vi "Packet.vi"(8 "error in (no error)":errorcluster, 9 "timeout ms (10000)":i32=10000, 11 "connection ID":refnum<k5>) -> (0 "error out":errorcluster, 1 "tx":T1, 2 "px":T2 {"Px16" format="%.2f"; "Px15" format="%.2f"; "Px14" format="%.2f"; "Px13" format="%.2f"; "Px12" format="%.2f"; "Px11" format="%.2f"; "Px10" format="%.2f"; "Px9" format="%.2f"; "Px8" format="%.2f"; "Px7" format="%.2f"; "Px6" format="%.2f"; "Px5" format="%.2f"; "Px4" format="%.2f"; "Px3" format="%.2f"; "Px2" format="%.2f"; "Px1" format="%.2f"}, 3 "connection ID out":refnum<k5>, 4 "frame":u32, 5 "status":string)   [LabVIEW 2019]
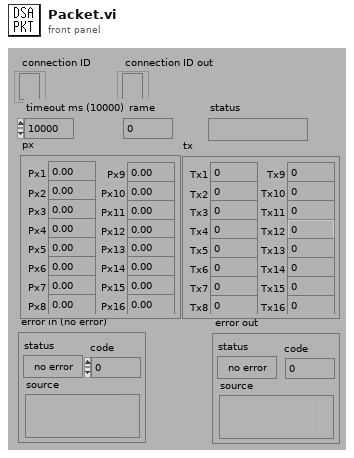
[diagram p1: front panel]
types:
  T1 = cluster{"Tx1":i16, "Tx2":i16, "Tx3":i16, "Tx4":i16, "Tx5":i16, "Tx6":i16, "Tx7":i16, "Tx8":i16, "Tx9":i16, "Tx10":i16, "Tx11":i16, "Tx12":i16, "Tx13":i16, "Tx14":i16, "Tx15":i16, "Tx16":i16}
  T2 = cluster{"Px1":sgl, "Px2":sgl, "Px3":sgl, "Px4":sgl, "Px5":sgl, "Px6":sgl, "Px7":sgl, "Px8":sgl, "Px9":sgl, "Px10":sgl, "Px11":sgl, "Px12":sgl, "Px13":sgl, "Px14":sgl, "Px15":sgl, "Px16":sgl}
  T3 = enum16{"Standard", "Buffered", "CRLF", "Immediate"}
  T4 = cluster{"[0]":i16, "[1]":i16, "[2]":i16, "[3]":i16, "[4]":i16, "[5]":i16, "[6]":i16, "[7]":i16, "[8]":i16, "[9]":i16, "[10]":i16, "[11]":i16, "[12]":i16, "[13]":i16, "[14]":i16, "[15]":i16}
  T5 = cluster{"[0]":sgl, "[1]":sgl, "[2]":sgl, "[3]":sgl, "[4]":sgl, "[5]":sgl, "[6]":sgl, "[7]":sgl, "[8]":sgl, "[9]":sgl, "[10]":sgl, "[11]":sgl, "[12]":sgl, "[13]":sgl, "[14]":sgl, "[15]":sgl}
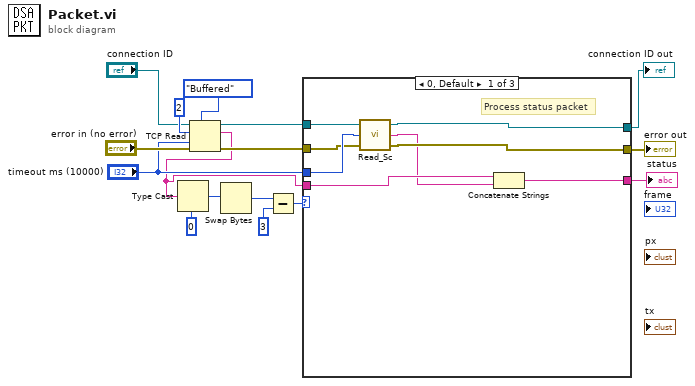
[diagram p0: block diagram]
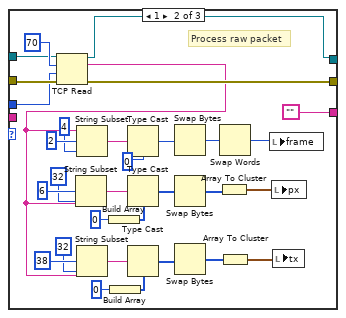
[diagram p2: hidden frame]
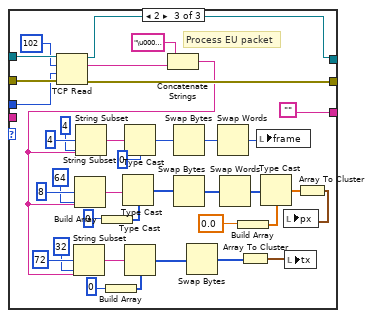
[diagram p3: hidden frame]
diagram:
  n1 = TCP Read(connection ID="connection ID", bytes to read=2, error in (no error)="error in (no error)", 7:T3."Buffered" ("mode (standard)"), 9:"timeout ms (10000)") -> (connection ID out=w14:refnum<k5>, data out=w1:string, error out=w13:errorcluster)
  n2 = Type Cast(type=u16 0, x=w1) -> (*(type *) &x=w10:u16)
  n3 = Swap Bytes(anything=w10) -> (byte swapped=w8:u16)
  n4 = Subtract(x=w8, y=u16 3) -> (x-y=w6:u16)
  n5 = case shown="0, Default" w6 {
    tunnel: w14 -> [w21 w54 w92]
    tunnel: w13 -> [w19 w53 w91]
    tunnel: [w18 w42 w81] -> w12
    tunnel: "timeout ms (10000)" -> [w20 w31 w61]
    tunnel: [w23 "" ""] -> w3
    tunnel: [w22 w26 w56] -> w2
    tunnel: w1 -> [w24 _ _]
    frame 0, Default {
      # "Process status packet"
      n6 = call "Read_Sc.vi"("error in (no error)"=w19, "timeout ms (10000)"=w20, "connection ID"=w21) -> ("error out"=w18:errorcluster, "data out"=w17:string, "connection ID out"=w22:refnum<k5>)
      n7 = Concatenate Strings(w24, w17) -> (w23:string)
    }
    frame 1 {
      # "Process raw packet"
      n8 = TCP Read(connection ID=w54, bytes to read=70, error in (no error)=w53, 9:w31) -> (connection ID out=w26:refnum<k5>, data out=w25:string, error out=w42:errorcluster)  [unwired: 1 in]
      n9 = String Subset(string=w25, offset (0)=6, length (rest)=32) -> (substring=w47:string)
      n10 = String Subset(string=w25, offset (0)=2, length (rest)=4) -> (substring=w40:string)
      n11 = String Subset(string=w25, offset (0)=38, length (rest)=32) -> (substring=w35:string)
      n12 = Build Array(i16 0) -> (w44:i16[])
      n13 = Build Array(i16 0) -> (w50:i16[])
      n14 = Type Cast(type=u32 0, x=w40) -> (*(type *) &x=w41:u32)
      n15 = Type Cast(type=w44, x=w47) -> (*(type *) &x=w48:i16[])
      n16 = Type Cast(type=w50, x=w35) -> (*(type *) &x=w34:i16[])
      n17 = Swap Bytes(anything=w41) -> (byte swapped=w37:u32)
      n18 = Swap Bytes(anything=w48) -> (byte swapped=w32:i16[])
      n19 = Swap Bytes(anything=w34) -> (byte swapped=w33:i16[])
      n20 = Array To Cluster(array=w32) -> (cluster=w29:T4)
      n21 = Swap Words(1:w37) -> (0:w30:u32)
      n22 = Array To Cluster(array=w33) -> (cluster=w28:T4)
      n23 = local write "frame"(w30) -> ()
      n24 = local write "px"(w29) -> ()
      n25 = local write "tx"(w28) -> ()
    }
    frame 2 {
      # "Process EU packet"
      n26 = TCP Read(connection ID=w92, bytes to read=102, error in (no error)=w91, 9:w61) -> (connection ID out=w56:refnum<k5>, data out=w88:string, error out=w81:errorcluster)  [unwired: 1 in]
      n27 = Build Array(u32 0) -> (w75:u32[])
      n28 = Build Array(i16 0) -> (w85:i16[])
      n29 = Concatenate Strings("\u0005\u0000", w88) -> (w78:string)
      n30 = String Subset(string=w78, offset (0)=72, length (rest)=32) -> (substring=w74:string)
      n31 = String Subset(string=w78, offset (0)=8, length (rest)=64) -> (substring=w68:string)
      n32 = String Subset(string=w78, offset (0)=4, length (rest)=4) -> (substring=w71:string)
      n33 = Type Cast(type=w75, x=w68) -> (*(type *) &x=w67:u32[])
      n34 = Type Cast(type=u32 0, x=w71) -> (*(type *) &x=w70:u32)
      n35 = Type Cast(type=w85, x=w74) -> (*(type *) &x=w73:i16[])
      n36 = Swap Bytes(anything=w70) -> (byte swapped=w69:u32)
      n37 = Swap Bytes(anything=w67) -> (byte swapped=w66:u32[])
      n38 = Swap Bytes(anything=w73) -> (byte swapped=w72:i16[])
      n39 = Swap Words(1:w69) -> (0:w60:u32)
      n40 = Swap Words(1:w66) -> (0:w65:u32[])
      n41 = Build Array(sgl 0.0) -> (w64:sgl[])
      n42 = Array To Cluster(array=w72) -> (cluster=w58:T4)
      n43 = local write "frame"(w60) -> ()
      n44 = Type Cast(type=w64, x=w65) -> (*(type *) &x=w63:sgl[])
      n45 = local write "tx"(w58) -> ()
      n46 = Array To Cluster(array=w63) -> (cluster=w59:T5)
      n47 = local write "px"(w59) -> ()
    }
  }
  "error out" <- w12
  "connection ID out" <- w2
  "status" <- w3
